vi "查询最早记录时间.vi"(11 "DB 引用":T1) -> (0 "error out":errorcluster, 3 "最小记录时间":timestamp, 4 "数据库连接引用out":T1)   [LabVIEW 2017]
uses:
  <vilib>/addons/database/Connection.llb/Conn ObjectReference.ctl
  <vilib>/addons/database/NI_Database_API.lvlib
panel:
  out "字符串":string
  out "各表最早记录时间":string[](array[string])
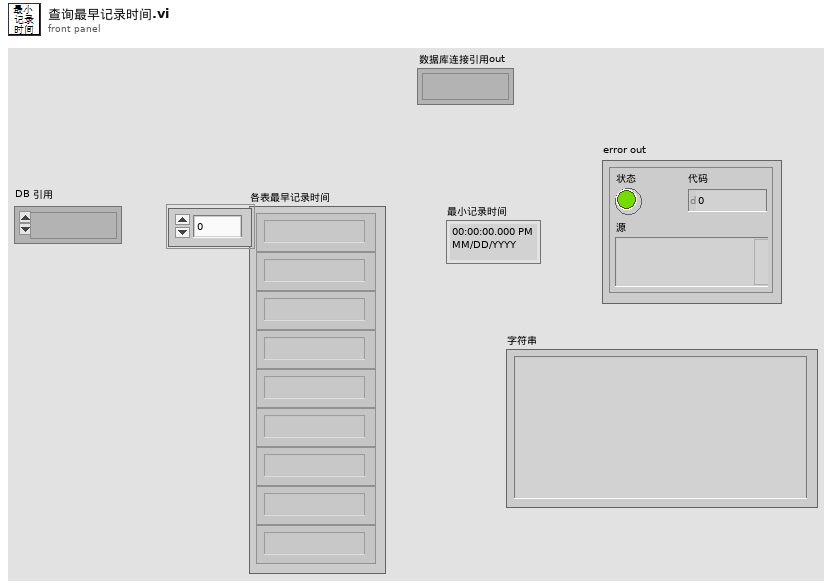
[diagram p1: front panel]
types:
  T1 = typedef "NI_Database_API.lvlib/Conn ObjectReference.ctl" = refnum<k1>
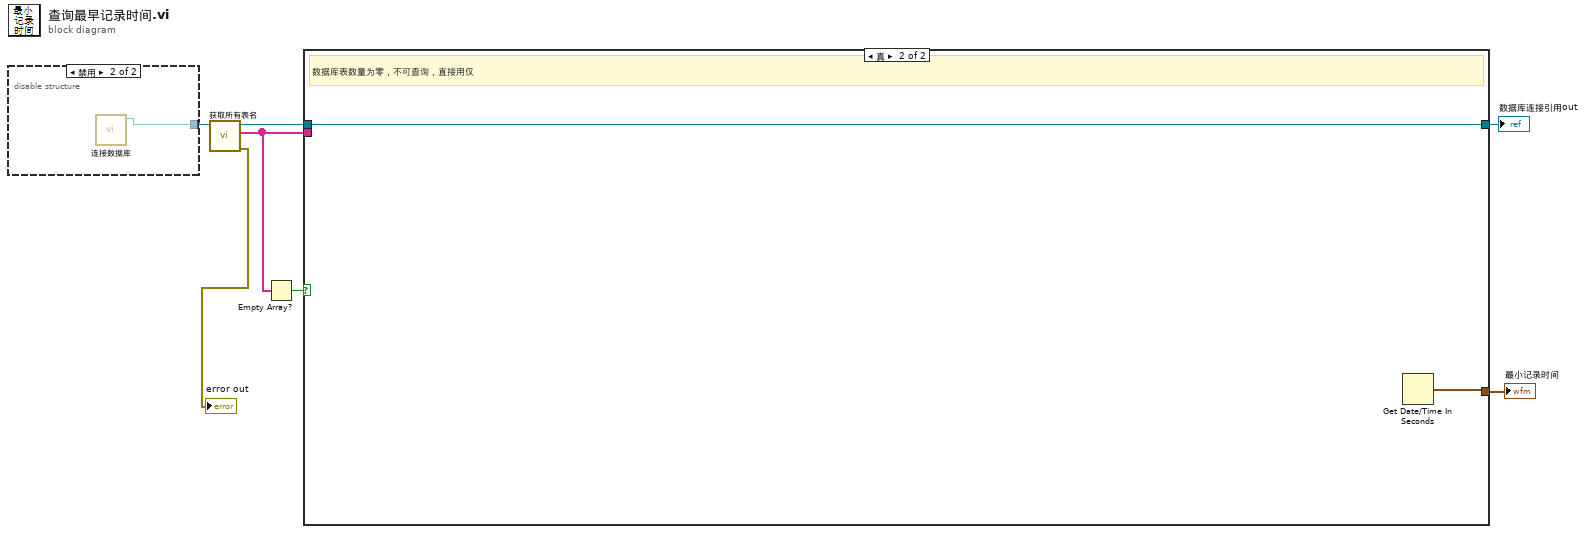
[diagram p0: block diagram]
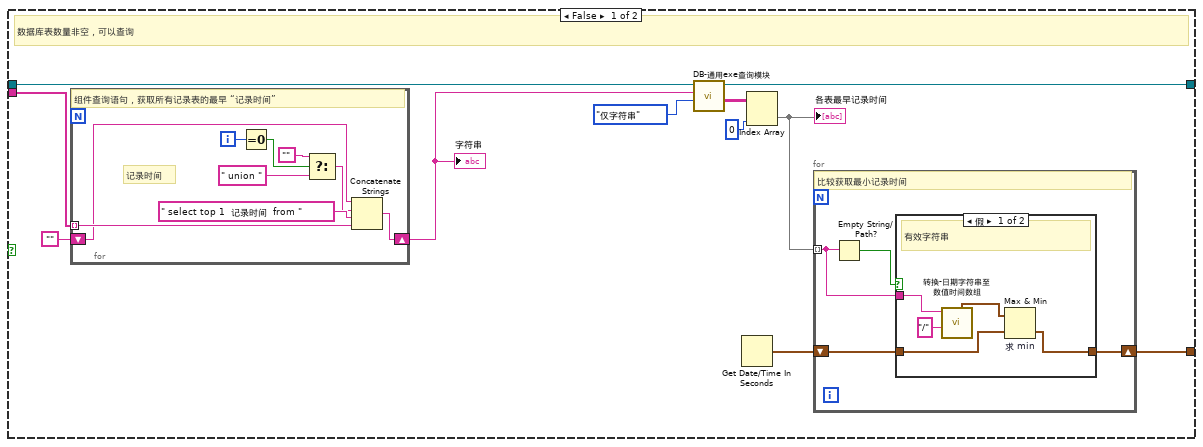
[diagram p2: hidden frame]
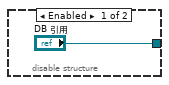
[diagram p4: hidden frame]
diagram:
  n1 = disable-structure shown="禁用" {
    disable-tunnel: ["DB 引用" w9] -> w7
    frame Enabled {
    }
    frame Disabled {
      n2 = call "连接数据库.vi"() -> ("connection reference"=w9:T1)  [unwired: 10 in, 1 out]
    }
  }
  n3 = call "获取所有表名.vi"("数据库连接引用 i"=w7) -> ("error out"=→"error out":errorcluster, "表名"=w4:string[], "数据库连接引用 o"=w6:T1)  [unwired: 8 in]
  n4 = Empty Array?(array=w4) -> (empty?=w3:bool)
  n5 = case shown="真" w3 {
    tunnel: w6 -> [w16 w40]
    tunnel: [w12 w41] -> w5
    tunnel: w4 -> [w11 _]
    tunnel: [w10 w40] -> w1
    frame False {
      # "数据库表数量非空，可以查询"
      n6 = for {
        tunnel: w11 -> [w38] mode=indexing
        shift-right: [w31] -> w17
        shift-left: "" -> [w32]
        i -> [w37]
        # "记录时间"
        # "组件查询语句，获取所有记录表的最早 “记录时间”"
        n7 = Equal To 0?(x=w37) -> (x = 0?=w36:bool)
        n8 = Select(t="", s=w36, f=" union " ("SQL query")) -> (s? t:f=w33:string)
        n9 = Concatenate Strings(w32, w33, " select top 1  记录时间  from " ("SQL query"), w38) -> (w31:string)
      }
      "字符串" <- w17
      n10 = call "DB-通用exe查询模块.vi"("解析模式"=enum16{"仅数值", "仅字符串", "数值与字符串"}."仅字符串", "SQL query"=w17, "数据库连接引用"=w16) -> ("字符串数据"=w19:string[][], "数据库连接引用out"=w10:T1)  [unwired: 4 in, 3 out]
      n11 = Get Date/Time In Seconds() -> (seconds since 1Jan1904=w13:timestamp)
      n12 = Index Array(array=w19, index (col)=0 ("禁用的索引 (列)")) -> (element=w14:string[])  [unwired: 1 in]
      "各表最早记录时间" <- w14
      n13 = for {
        tunnel: w14 -> [w23] mode=indexing
        shift-right: [w21] -> w12
        shift-left: w13 -> [w22]
        # "比较获取最小记录时间"
        n14 = Empty String/Path?(string/path=w23) -> (empty?=w24:bool)
        n15 = case shown="假" w24 {
          tunnel: w23 -> [w29 _]
          tunnel: w22 -> [w28 w30]
          tunnel: [w26 w30] -> w21
          frame False {
            # "有效字符串"
            n16 = call "转换-日期字符串至数值时间数组.vi"("分隔符（/）"="/", "日期时间（或仅日期）字符串"=w29) -> ("时间标识"=w27:timestamp)  [unwired: 5 in, 4 out]
            n17 = Max & Min "求 min"(x=w27, y=w28) -> (min(x,y)=w26:timestamp)  [unwired: 1 out]
          }
          frame True {
            # "无效"
          }
        }
      }
    }
    frame True {
      # "数据库表数量为零，不可查询，直接用仅"
      n18 = Get Date/Time In Seconds() -> (seconds since 1Jan1904=w41:timestamp)
    }
  }
  "最小记录时间" <- w5
  "数据库连接引用out" <- w1
